vi "PD500 - DC Bus Test.vi"(8 "error in (no error)":errorcluster, 11 "Board Selector":T1) -> (0 "error out":errorcluster, 1 "INVB":dbl[](array[numeric]), 2 "INVA":dbl[](array[numeric]))   [LabVIEW 2022 SP3]
uses:
  Serial Board Com/Board Select.ctl
  Serial Board Com/ADCSelector GB.ctl
  Serial Board Com/ADCSelector BB.ctl
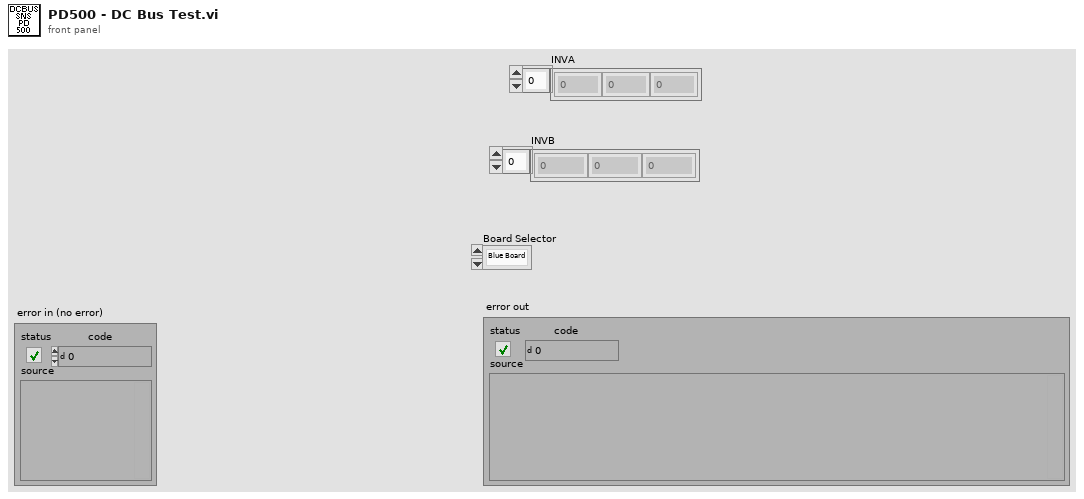
[diagram p1: front panel]
types:
  T1 = typedef "Board Select.ctl" = enum16{"Blue Board", "Green Board"}
  T2 = cluster{"Delay Before Read":dbl, "Vdc Cmd":dbl, "Relay Command":bool[]}[]
  T3 = typedef "ADCSelector BB.ctl" = enum16{"INVA_ISENSE_U", "INVA_ISENSE_V", "INVA_ISENSE_W", "INVA_UDC", "INVA_TEMP", "HB_TEMP", "AUXB_TEMP", "VLINE_AB", "VLINE_BC", "VLINE_CA", "VSENSE_POS_24V", "VSENSE_POS_5V", "VSENSE_NEG_15V", "INVB_ISENSE_U", "INV_B_ISENSEV", "INVB_ISENSE_W", "INVB_UDC", "INVB_TEMP", "AUXA_TEMP", "AUXC_TEMP", "VOUT_AB", "VOUT_BC", "VOUT_CA", "VSENSE_POS_15V", "VSENSE_POS_3P3V", "TEST_POINT"}
  T4 = typedef "ADCSelector GB.ctl" = enum16{"INVA_ISENSE_U", "INVA_ISENSE_V", "INVA_ISENSE_W", "INVA_UDC", "INVA_TEMP", "HB_ISENSE", "AUX_ISENSE_U", "AUX_ISENSE_V", "AUX_ISENSE_W", "VLINE_AB", "VLINE_BC", "VLINE_CA", "REF_1P5V", "VSENSE_POS_24V", "VSENSE_POS_5V", "VSENSE_NEG_15V", "TEST_POINT", "INVB_ISENSE_U", "INVB_ISENSE_V", "INVB_ISENSE_W", "INVB_UDC", "INVB_TEMP", "HB_TEMP", "AUXA_TEMP", "AUXB_TEMP", "AUXC_TEMP", "VOUT_AB", "VOUT_BC", "VOUT_CA", "REF_2P5V", "VSENSE_POS_15V", "VSENSE_POS_3P3V", "NET_ANALYZER"}
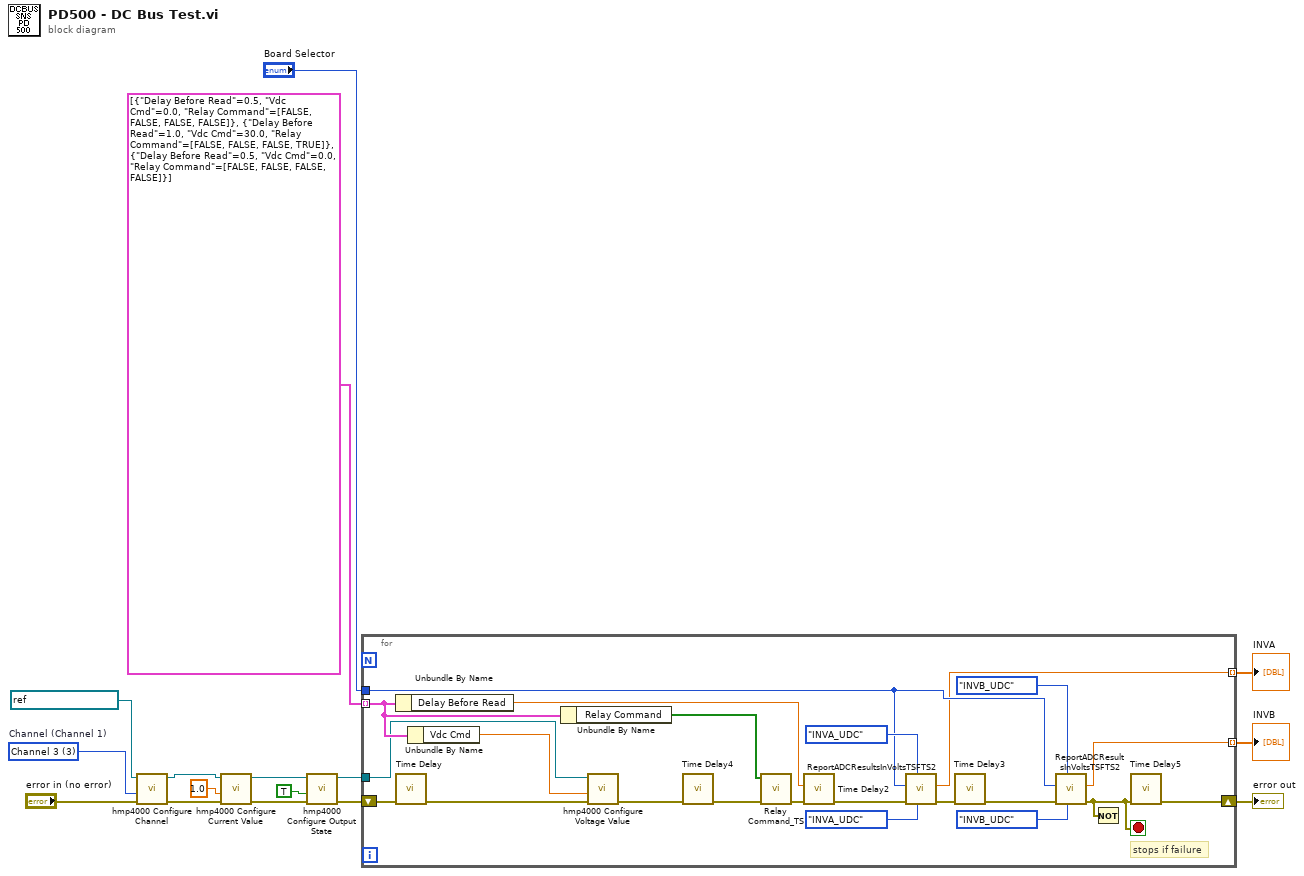
[diagram p0: block diagram]
diagram:
  w13 = 3 items=["Channel 1"=1, "Channel 2"=2, "Channel 3"=3, "Channel 4"=4]  # Channel (Channel 1)
  n1 = call <instrlib>:"hmp4000 Configure Channel.vi"("error in (no error)"="error in (no error)", "Channel (Channel 1)"=w13, "VISA resource name"=refnum<visa-resource-name> "HMP4040_FTS2" ("HMP4040 IN")) -> ("error out"=w9:errorcluster, "VISA resource name out"=w6:refnum<visa-resource-name>)  [unwired: 7 in]
  n2 = call <instrlib>:"hmp4000 Configure Current Value.vi"("error in (no error)"=w9, "Current (0.0)"=1.0, "VISA resource name"=w6) -> ("error out"=w8:errorcluster, "VISA resource name out"=w5:refnum<visa-resource-name>)  [unwired: 7 in]
  n3 = call <instrlib>:"hmp4000 Configure Output State.vi"("error in (no error)"=w8, "Output State (Off)"=TRUE, "VISA resource name"=w5) -> ("error out"=w11:errorcluster, "VISA resource name out"=w4:refnum<visa-resource-name>)  [unwired: 7 in]
  n4 = for {
    shift-right: [w17] -> w15
    shift-left: w11 -> [w30]
    tunnel: T2 [{"Delay Before Read"=0.5, "Vdc Cmd"=0.0, "Relay Command"=[FALSE, FALSE, FALSE, FALSE]}, {"Delay Before Read"=1.0, "Vdc Cmd"=30.0, "Relay Command"=[FALSE, FALSE, FALSE, TRUE]}, {"Delay Before Read"=0.5, "Vdc Cmd"=0.0, "Relay Command"=[FALSE, FALSE, FALSE, FALSE]}] -> [w34] mode=indexing
    tunnel: "Board Selector" -> [w31]
    tunnel: w4 -> [w27]
    tunnel: [w26] -> w3 mode=indexing
    tunnel: [w25] -> w2 mode=indexing
    stop <- w18 stop-if-true
    # "stops if failure"
    n5 = Unbundle By Name(w34) -> ("Delay Before Read"=w37:dbl)
    n6 = call "Time Delay"("error in (no error)"=w30) -> ("error out"=w29:errorcluster)  [unwired: 10 in]
    n7 = Unbundle By Name(w34) -> ("Vdc Cmd"=w36:dbl)
    n8 = Unbundle By Name(w34) -> ("Relay Command"=w28:bool[])
    n9 = call <instrlib>:"hmp4000 Configure Voltage Value.vi"("error in (no error)"=w29, "Voltage (0.0)"=w36, "VISA resource name"=w27) -> ("error out"=w20:errorcluster)  [unwired: 7 in, 1 out]
    n10 = call "Time Delay4"("error in (no error)"=w20) -> ("error out"=w19:errorcluster)  [unwired: 10 in]
    n11 = call "Relay Command_TS.vi"("error in (no error)"=w19, "Relay Command"=w28) -> ("error out"=w35:errorcluster)  [unwired: 8 in, 1 out]
    n12 = call "Time Delay2"("error in (no error)"=w35, "Delay Time (s)"=w37) -> ("error out"=w38:errorcluster)  [unwired: 9 in]
    n13 = call "ReportADCResultsInVoltsTSFTS2.vi"("Blue Board Enum"=ADCSelector_BB."INVA_UDC", "Green Board Enum"=ADCSelector_GB."INVA_UDC" ("Enum"), "error in (no error)"=w38, "Board Selector"=w31) -> ("error out"=w22:errorcluster, "Result"=w26:dbl)  [unwired: 4 in, 2 out]
    n14 = call "Time Delay3"("error in (no error)"=w22) -> ("error out"=w21:errorcluster)  [unwired: 10 in]
    n15 = call "ReportADCResultsInVoltsTSFTS2.vi"("Blue Board Enum"=ADCSelector_BB."INVB_UDC", "Green Board Enum"=ADCSelector_GB."INVB_UDC" ("Enum"), "error in (no error)"=w21, "Board Selector"=w31) -> ("error out"=w18:errorcluster, "Result"=w25:dbl)  [unwired: 4 in, 2 out]
    n16 = Not(x=w18) -> ()  [unwired: 1 out]
    n17 = call "Time Delay5"("error in (no error)"=w18) -> ("error out"=w17:errorcluster)  [unwired: 10 in]
  }
  "error out" <- w15
  "INVA" <- w3
  "INVB" <- w2
